vi "Orifice Flow Calculation For Air Iso5167.vi"(0 "RH":dbl min=0.0 max=100.0, 1 "Orifice Diameter":dbl[unit], 2 "Gas Temperature":dbl[unit]=10.0 min=10.0 max=95.0, 3 "P1\n(Presure After Fan &\n before Orifice)":dbl[unit]=80000.0 min=80000.0 max=120000.0, 4 "Pipe Diameter (mm)":dbl[unit], 5 "Delta P\n(Presure Made By Orifice)":dbl[unit]) -> (6 "Mass Flow (Orifice) (Kg/h)":dbl[unit], 7 "Iteration Volumetric Flow \n(Orifice) (m^3/s)":dbl[unit], 8 "Air Flow":bool)   [LabVIEW 2018]
panel:
  out "Mass Flow (Orifice) (Kg/h)":dbl[unit](knob)
  out "Mass Flow (Orifice) (Kg/s)":dbl[unit]
  out "ReD":dbl
  out "Gas Viscosity\nof Humid Air":dbl[unit]
  out "Pipe Velocity (m/s)":dbl[unit]
  out "Pipe Area (m^2)":dbl[unit]
  out "Throat Velocity (m/s)":dbl[unit]
  out "Throat Area (m^2)":dbl[unit]
  out "Beta":dbl
  out "Pipe Diameter (inch)":dbl[unit]
  out "orifice coefficient":dbl
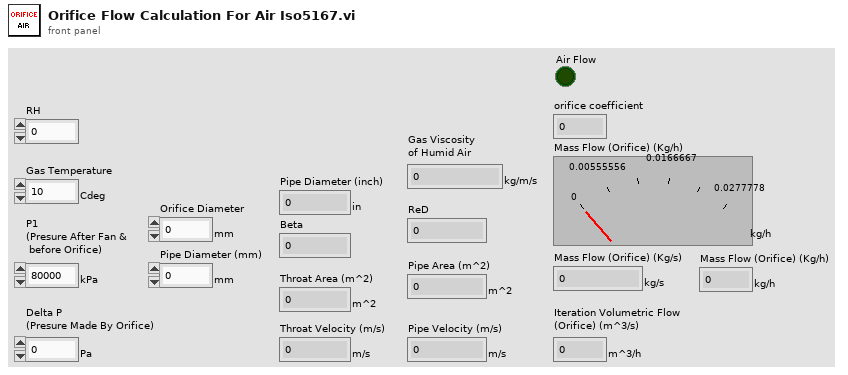
[diagram p1: front panel]
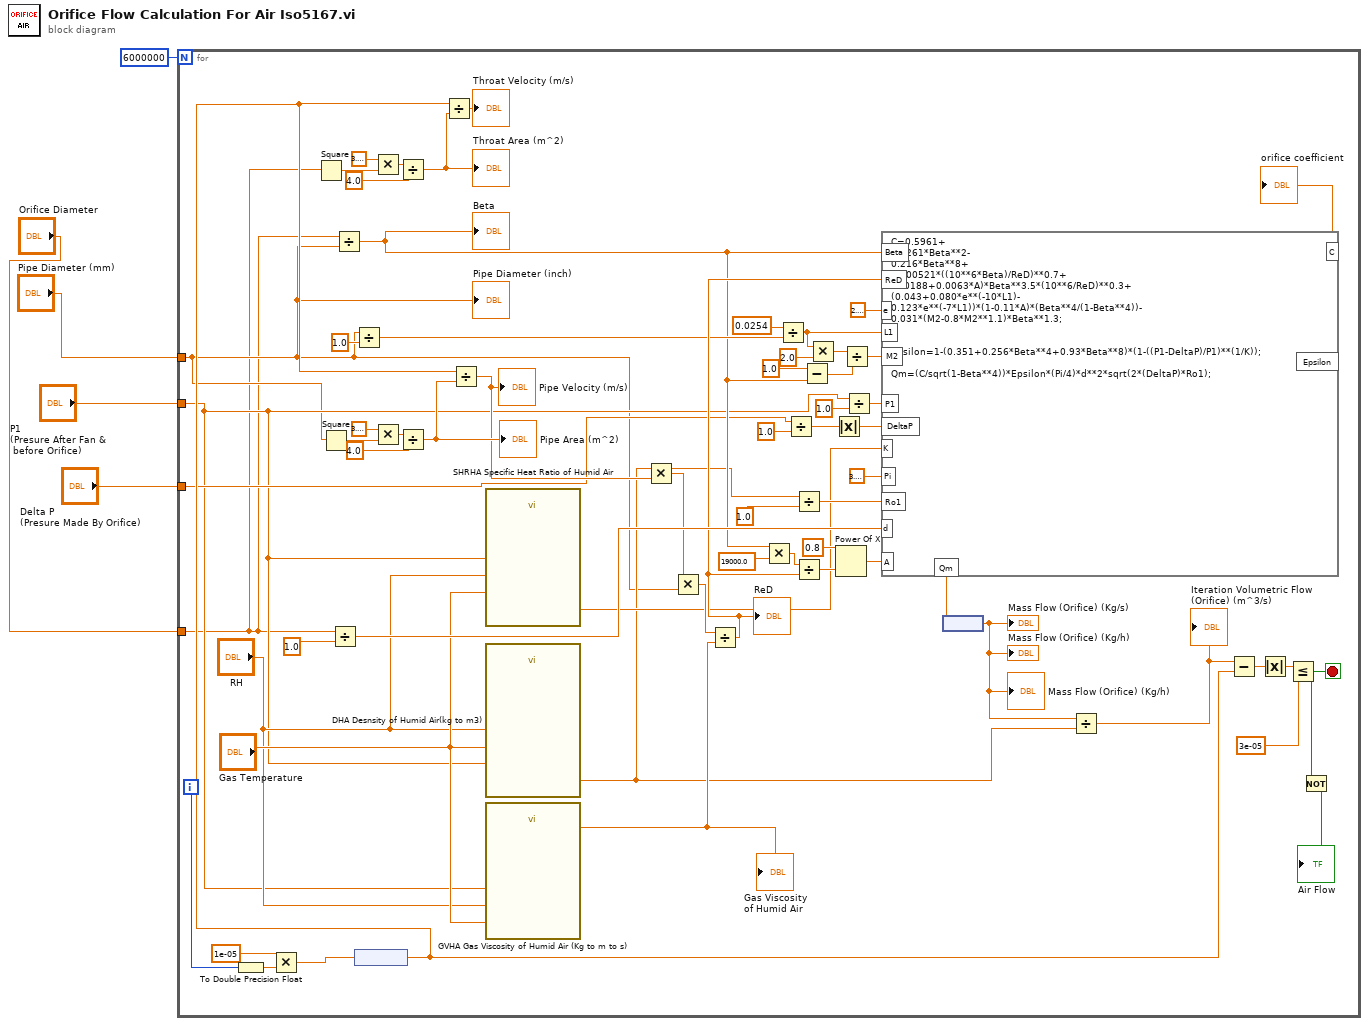
[diagram p0: block diagram]
diagram:
  n1 = for {
    N: 6000000 -> [_]
    tunnel: "Delta P\n(Presure Made By Orifice)" -> [w12]
    tunnel: "P1\n(Presure After Fan &\n before Orifice)" -> [w11]
    tunnel: "Pipe Diameter (mm)" -> [w10]
    tunnel: "Orifice Diameter" -> [w9]
    i -> [w27]
    stop <- w13 stop-if-true
    n2 = To Double Precision Float(number=w27) -> (double precision float=w29:dbl)
    n3 = Multiply(x=1e-05, y=w29) -> (x*y=w8:dbl)
    n4 = Square(x=w9) -> (x^2=w63:dbl[unit])
    n5 = Square(x=w10) -> (x^2=w59:dbl[unit])
    n6 = Divide(x=w9, y=dbl[unit] 1.0) -> (x/y=w55:dbl)
    n7 = Divide(x=w9, y=w10) -> (x/y=w32:dbl)
    "Beta" <- w32
    n8 = Divide(x=w10, y=dbl[unit] 1.0) -> (x/y=w43:dbl)
    n9 = node(w8) -> (w26:dbl[unit])
    n10 = Multiply(x=3.141592653589793, y=w63) -> (x*y=w65:dbl[unit])
    n11 = Multiply(x=3.141592653589793, y=w59) -> (x*y=w61:dbl[unit])
    n12 = Divide(x=w65, y=4.0) -> (x/y=w67:dbl[unit])
    "Throat Area (m^2)" <- w67
    n13 = Divide(x=w61, y=4.0) -> (x/y=w58:dbl[unit])
    "Pipe Area (m^2)" <- w58
    n14 = Divide(x=w26, y=w67) -> (x/y=→"Throat Velocity (m/s)":dbl[unit])
    n15 = Divide(x=w26, y=w58) -> (x/y=w51:dbl[unit])
    "Pipe Velocity (m/s)" <- w51
    n16 = call "SHRHA Specific Heat Ratio of Humid Air.vi"("Gas Presure"=w11, "Tceg"="Gas Temperature", "RH"="RH") -> ("SHRHA"=w31:dbl)
    n17 = call "DHA Desnsity of Humid Air(kg to m3).vi"("Total Pressure of Humid Air"=w11, "Tceg"="Gas Temperature", "RH"="RH") -> ("DHA"=w15:dbl[unit])
    n18 = call "GVHA Gas Viscosity of Humid Air (Kg to m to s).vi"("Gas Presure"=w11, "Tceg"="Gas Temperature", "RH"="RH") -> ("Gas Viscosity Of  Humid Air"=w19:dbl[unit])
    "Gas Viscosity\nof Humid Air" <- w19
    n19 = Multiply(x=w15, y=w51) -> (x*y=w52:dbl[unit])
    n20 = Multiply(x=w52, y=w10) -> (x*y=w53:dbl[unit])
    n21 = Divide(x=w53, y=w19) -> (x/y=w48:dbl)
    "ReD" <- w48
    n22 = Multiply(x=w32, y=19000.0) -> (x*y=w49:dbl)
    n23 = Divide(x=0.0254, y=w43) -> (x/y=w42:dbl)
    n24 = Divide(x=w12, y=dbl[unit] 1.0) -> (x/y=w16:dbl)
    n25 = Divide(x=w15, y=dbl[unit] 1.0) -> (x/y=w37:dbl)
    n26 = Divide(x=w49, y=w48) -> (x/y=w47:dbl)
    n27 = Subtract(x=1.0, y=w32) -> (x-y=w33:dbl)
    n28 = Multiply(x=w42, y=2.0) -> (x*y=w40:dbl)
    n29 = Absolute Value(x=w16) -> (abs(x)=w7:dbl)
    n30 = Power Of X(1:w47, 2:0.8 ("y")) -> (0:w45:dbl)
    n31 = Divide(x=w40, y=w33) -> (x/y=w38:dbl)
    n32 = Divide(x=w11, y=dbl[unit] 1.0) -> (x/y=w22:dbl)
    n33 = formula code="C=0.5961+\n0.0261*Beta**2-\n0.216*Beta**8+\n0.000521*((10**6*Beta)/ReD)**0.7+\n(0.0188+0.0063*A)*Beta**3.5*(10**6/ReD)**0.3+\n(0.043+0.080*e**(-10*L1)-\n0.123*e**(-7*L1))*(1-0.11*A)*(Beta**4/(1-Beta**4))-\n0.031*(M2-0.8*M2**1.1)*Beta**1.3;\n\n\nEpsilon=1-(0.351+0.256*Beta**4+0.93*Beta**8)*(1-((P1-DeltaP)/P1)**(1/K));\n\nQm=(C/sqrt(1-Beta**4))*Epsilon*(Pi/4)*d**2*sqrt(2*(DeltaP)*Ro1);"("Beta"=w32, "ReD"=w48, "A"=w45, "e"=2.718281828459045, "L1"=w42, "M2"=w38, "P1"=w22, "DeltaP"=w7, "K"=w31, "Pi"=3.141592653589793, "Ro1"=w37, "d"=w55) -> ("C"=→"orifice coefficient":dbl, "Qm"=w35:dbl)  [unwired: 1 out]
    n34 = node(w35) -> (w30:dbl[unit])
    "Mass Flow (Orifice) (Kg/s)" <- w30
    "Mass Flow (Orifice) (Kg/h)" <- w30
    "Mass Flow (Orifice) (Kg/h)" <- w30
    n35 = Divide(x=w30, y=w15) -> (x/y=w18:dbl[unit])
    "Iteration Volumetric Flow \n(Orifice) (m^3/s)" <- w18
    n36 = Subtract(x=w18, y=w26) -> (x-y=w25:dbl[unit])
    n37 = Absolute Value(x=w25) -> (abs(x)=w24:dbl[unit])
    n38 = Less Or Equal?(x=w24, y=dbl[unit] 3e-05) -> (x <= y?=w13:bool)
    n39 = Not(x=w13) -> (.not. x?=→"Air Flow":bool)
    "Pipe Diameter (inch)" <- w10
  }
